vi "Shutdown Daemon.vi"(8 "error in":errorcluster, 11 "Serial Slave in":refnum<class "Serial Slave.lvclass">) -> (0 "error out":errorcluster)   [LabVIEW 2021, in "Serial Slave.lvclass"]
doc: "This provides an interface for the slave to shut down its protocol daemon."
uses:
  Serial Slave.lvclass
  Serial Slave.lvclass/Serial Slave.ctl
  Network Slave.lvclass
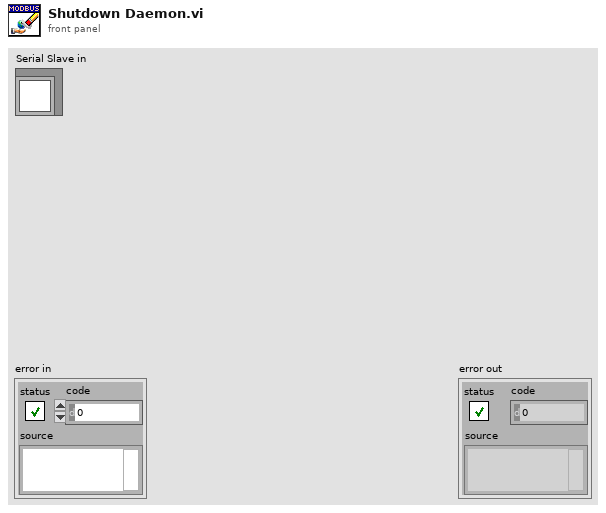
[diagram p1: front panel]
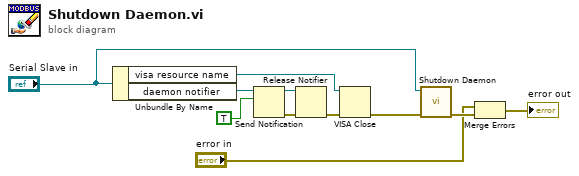
[diagram p0: block diagram]
diagram:
  n1 = Unbundle By Name("Serial Slave in") -> ("visa resource name"=w7:refnum<visa-resource-name>, "daemon notifier"=w8:refnum<notifier>)
  n2 = Send Notification(notification=TRUE, notifier=w8) -> (notifier out=w10:refnum<notifier>, error out=w9:errorcluster)  [unwired: 1 in]
  n3 = Release Notifier(notifier=w10, error in (no error)=w9) -> (error out=w6:errorcluster)  [unwired: 1 in, 2 out]
  n4 = VISA Close(VISA resource name=w7, error in (no error)=w6) -> (error out=w4:errorcluster)
  n5 = call-parent "Shutdown Daemon.vi"("error in"=w4, "network slave in"="Serial Slave in") -> ("error out"=w3:errorcluster)  [unwired: 9 in]
  n6 = Merge Errors("error in", w3) -> (→"error out":errorcluster)
